vi "Menue_Callback.vi"(8 "error in (no error)":errorcluster, 11 "MenueItem in":refnum<class "MenueItem.lvclass">) -> (0 "error out":errorcluster, 3 "MenueItem out":refnum<class "MenueItem.lvclass">)   [LabVIEW 2016, in "MenueItem.lvclass"]
uses:
  MenueItem.lvclass
  MenueItem.lvclass/MenueItem.ctl
  System.Windows.Forms
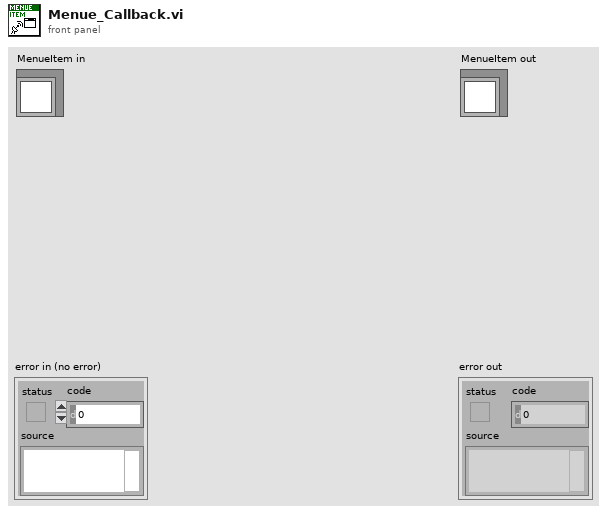
[diagram p1: front panel]
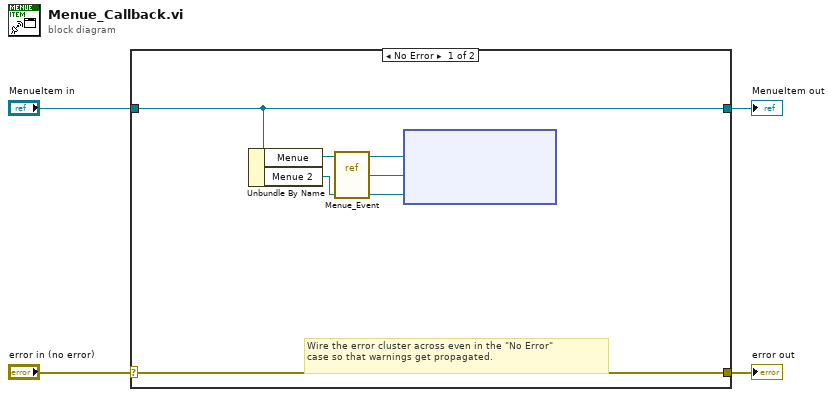
[diagram p0: block diagram]
diagram:
  n1 = case shown="No Error" "error in (no error)" {
    selector: "error in (no error)" -> [w9 w11]
    tunnel: [w9 w11] -> w3
    tunnel: [w8 w10] -> w1
    tunnel: "MenueItem in" -> [w8 w10]
    frame No Error {
      # "Wire the error cluster across even in the \"No Error\"\ncase so that warnings get propagated."
      n2 = Unbundle By Name(w8) -> ("Menue"=w7:refnum<k24>, "Menue 2"=w6:refnum<user-event>)
      n3 = vi-ref "Menue_Event.vi"() -> ("vi reference"=w5:refnum<vi>)
      n4 = node(w7, w5, w6) -> ()  [unwired: 2 in, 2 out]
    }
    frame Error {
    }
  }
  "error out" <- w3
  "MenueItem out" <- w1
